vi "armStatesLogic.vi"(10 "raiseArmButton":bool, 11 "lowerArmButton":bool) -> (3 "currentState":T1)   [LabVIEW 2018]
uses:
  Implementation/Manipulator Operations.ctl
  <vilib>/FRC Team #3937/Memory Library/memLib.lvlib
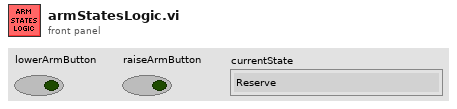
[diagram p1: front panel]
types:
  T1 = typedef "Manipulator Operations.ctl" = enum16{"Reserve", "Read Current", "Immediate", "LowerArm", "RaiseArm", "HoldingCover"}
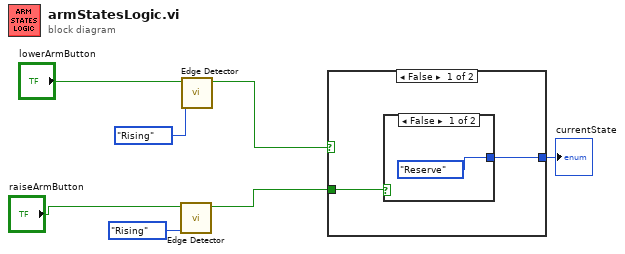
[diagram p0: block diagram]
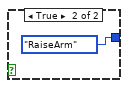
[diagram p2: hidden frame]
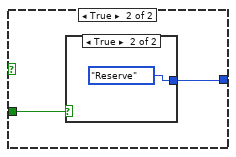
[diagram p3: hidden frame]
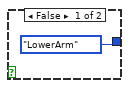
[diagram p4: hidden frame]
diagram:
  n1 = call <vilib>:"Edge Detector.vi"("Mode"=enum16{"Rising", "Falling", "Any"}."Rising", "Input"="raiseArmButton") -> ("Output"=w6:bool)  [unwired: 9 in]
  n2 = call <vilib>:"Edge Detector.vi"("Mode"=enum16{"Rising", "Falling", "Any"}."Rising", "Input"="lowerArmButton") -> ("Output"=w7:bool)  [unwired: 9 in]
  n3 = case shown="False" w7 {
    tunnel: w6 -> [w8 w13]
    tunnel: [w9 w12] -> w3
    frame False {
      n4 = case shown="False" w8 {
        tunnel: [Manipulator_Operations."Reserve" ("Enum") Manipulator_Operations."RaiseArm" ("Enum")] -> w9
        frame False {
        }
        frame True {
        }
      }
    }
    frame True {
      n5 = case shown="True" w13 {
        tunnel: [Manipulator_Operations."LowerArm" ("Enum") Manipulator_Operations."Reserve" ("Enum")] -> w12
        frame False {
        }
        frame True {
        }
      }
    }
  }
  "currentState" <- w3
